vi "ReadClipboard.vi"() -> (1 "Image Out":T1 {"Dialogs" format="%.0b"})   [LabVIEW 2024]
doc: "This VI loads an image from your computer's clipboard. For instance, if a user \"copies\" an image from a website into the computer's clipboard, that image data will be available to other VI's as an output from this VI."
uses:
  <userlib>/ImageProcessing/QTLIB_2595_LV86/QT_Image.ctl
panel:
  in  "Image":T1 {"Dialogs" format="%.0b"}
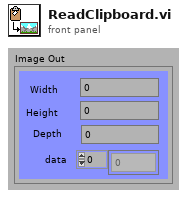
[diagram p1: front panel]
types:
  T1 = typedef "QT_Image.ctl" = cluster{"Width":i32, "Height":i32, "Depth":i32, "data":u8[], "Compressed data":u8[], "Color table":u32[], "Duration":i32, "Options":i32, "Timestamp":i32, "ID":i32, "Reserved":i32, "Dialogs":u32}
  T2 = typedef "LVRectTypeDef.ctl" = cluster{"left":i16, "top":i16, "right":i16, "bottom":i16}
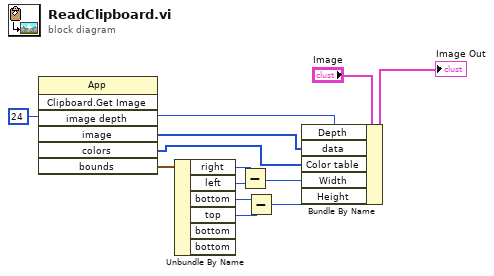
[diagram p0: block diagram]
diagram:
  w2 = 24 ("Image Depth")
  n1 = invoke class="App" method="Clipboard.Get Image"("image depth"=w2) -> ("image"=w3:u8[], "colors"=w4:u32[], "bounds"=w11:T2)  [unwired: 6 in, 4 out]
  n2 = Unbundle By Name(w11) -> ("right"=w9:i16, "left"=w10:i16, "bottom"=w6:i16, "top"=w7:i16)  [unwired: 2 out]
  n3 = Subtract(x=w9, y=w10) -> (x-y=w8:i16)
  n4 = Subtract(x=w6, y=w7) -> (x-y=w5:i16)
  n5 = Bundle By Name(cluster="Image", "Depth"=w2, "data"=w3, "Color table"=w4, "Width"=w8, "Height"=w5) -> (→"Image Out":T1)
